vi "draw.vi"(8 "error in (no error)":errorcluster, 9 "depth":dbl[unit], 10 "Image.lvclass":refnum<class "Image.lvclass">, 11 "RoiCollection in":refnum<class "RoiCollection.lvclass">) -> (0 "error out":errorcluster, 3 "RoiCollection out":refnum<class "RoiCollection.lvclass">)   [LabVIEW 2010, in "RoiCollection.lvclass"]
uses:
  RoiCollection.lvclass
  common/classes/Image/Image/Image.lvclass
  RoiCollection.lvclass/RoiCollection.ctl
  RoiGeneric/RoiGeneric.lvclass
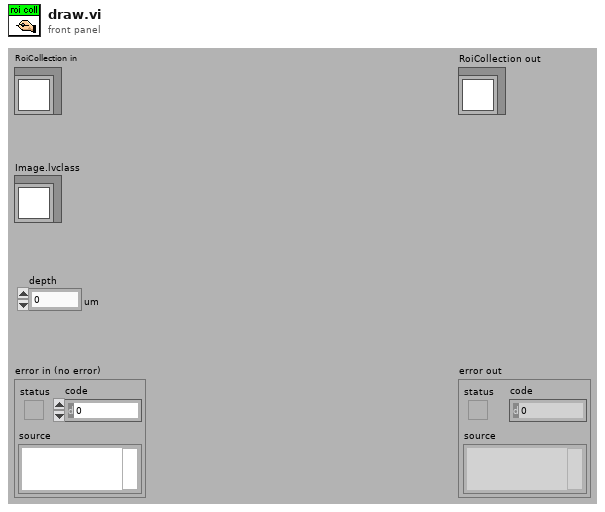
[diagram p1: front panel]
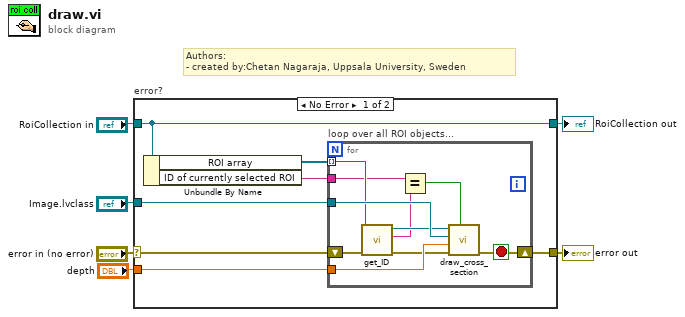
[diagram p0: block diagram]
diagram:
  # "Authors: \n- created by:Chetan Nagaraja, Uppsala University, Sweden"
  n1 = case "error?" shown="No Error" "error in (no error)" {
    selector: "error in (no error)" -> [w13 w25]
    tunnel: [w12 w25] -> w5
    tunnel: [w9 w24] -> w3
    tunnel: "RoiCollection in" -> [w9 w24]
    tunnel: "depth" -> [w11 _]
    tunnel: "Image.lvclass" -> [w10 _]
    frame No Error {
      n2 = Unbundle By Name(w9) -> ("ROI array"=w8:refnum<class "RoiGeneric.lvclass">[], "ID of currently selected ROI"=w7:string)
      n3 = for "loop over all ROI objects..." {
        tunnel: w11 -> [w23]
        tunnel: w10 -> [w22]
        tunnel: w8 -> [w18] mode=indexing
        shift-right: [w21] -> w12
        shift-left: w13 -> [w20]
        tunnel: w7 -> [w16]
        stop <- w21 stop-if-true
        n4 = call-dynamic "get_ID.vi"("error in (no error)"=w20, "RoiGeneric in"=w18) -> ("error out"=w19:errorcluster, "ID"=w15:string, "RoiGeneric out"=w17:refnum<class "RoiGeneric.lvclass">)  [unwired: 7 in]
        n5 = Equal?(x=w16, y=w15) -> (x = y?=w14:bool)
        n6 = call-dynamic "draw_cross_section.vi"("highlight?"=w14, "error in (no error)"=w19, "depth"=w23, "Image.lvclass"=w22, "RoiGeneric in"=w17) -> ("error out"=w21:errorcluster)  [unwired: 5 in, 1 out]
      }
    }
    frame Error {
    }
  }
  "error out" <- w5
  "RoiCollection out" <- w3
